vi "RunOperation.vi"(10 "Inputs":string[](array[string]), 11 "Restore in":refnum<class "Restore.lvclass">) -> (1 "Output/Failure":string, 2 "CLI Process Return Code":i32, 3 "Restore out":refnum<class "Restore.lvclass">)   [LabVIEW 2017, in "Restore.lvclass"]
uses:
  Restore.lvclass
  Restore.lvclass/Restore.ctl
  <vilib>/JKI/VIPM API/VIPM API_vipm_api.lvlib
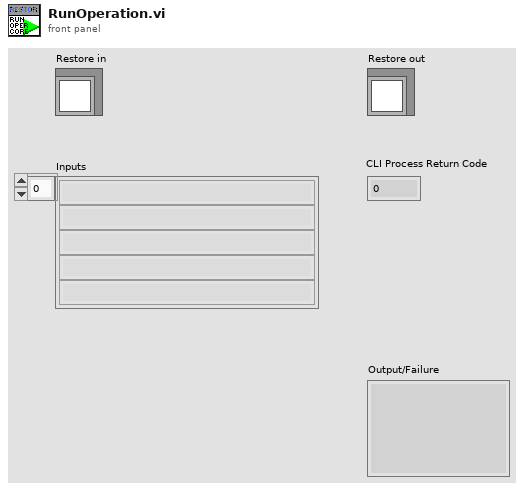
[diagram p1: front panel]
types:
  T1 = typedef "VIPM API_vipm_api.lvlib/LabVIEW Target Info Cluster_vipm_api.ctl" = cluster{"Version":string, "Connection Tested":bool, "Disabled":bool}
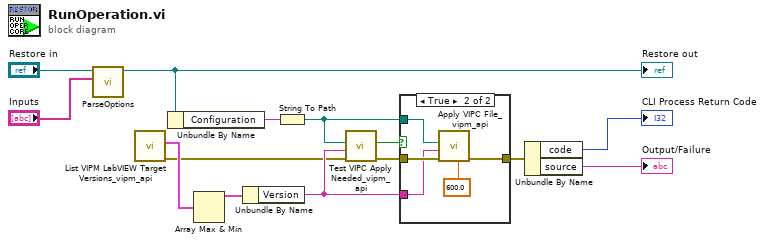
[diagram p0: block diagram]
diagram:
  n1 = call "ParseOptions.vi"("Options"="Inputs", "Restore in"="Restore in") -> ("Restore out"=w12:refnum<class "Restore.lvclass">)  [unwired: 8 in, 1 out]
  "Restore out" <- w12
  n2 = call <vilib>:"List VIPM LabVIEW Target Versions_vipm_api.vi"() -> ("error out"=w1:errorcluster, "LabVIEW Target Info"=w4:T1[])  [unwired: 10 in]
  n3 = Unbundle By Name(w12) -> ("Configuration"=w11:string)
  n4 = Array Max & Min(array=w4) -> (max value=w3:T1)  [unwired: 3 out]
  n5 = Unbundle By Name(w3) -> ("Version"=w2:string)
  n6 = String To Path(string=w11) -> (path=w5:path)
  n7 = call <vilib>:"Test VIPC Apply Needed_vipm_api.vi"("error in (no error)"=w1, "LabVIEW Version (use vipc version)"=w2, "VIPC File Path"=w5) -> ("error out"=w7:errorcluster, "Need to Apply?"=w6:bool)  [unwired: 6 in, 1 out]
  n8 = case shown="True" w6 {
    tunnel: [w15 w19] -> w10
    tunnel: w7 -> [w15 w18]
    tunnel: w5 -> [_ w17]
    tunnel: w2 -> [_ w16]
    frame False {
    }
    frame True {
      n9 = call <vilib>:"Apply VIPC File_vipm_api.vi"("Timeout in seconds (0: no timeout)"=600.0, "error in (no error)"=w18, "LabVIEW Version"=w16, "VIPC File"=w17) -> ("error out"=w19:errorcluster)  [unwired: 7 in]
    }
  }
  n10 = Unbundle By Name(w10) -> ("code"=→"CLI Process Return Code":i32, "source"=→"Output/Failure":string)
